vi "getDataByName.vi"(2 "Data Entry Name":string, 3 "Property Array In":T1[](array[typedef])) -> (0 "Value":string[](array[string]), 1 "Entity Type":string[](array[string]))   [LabVIEW 2016]
uses:
  typeDefs/singleDXFobject.ctl
  typeDefs/singleDXFvar.ctl
  dxf typedef.lvlib
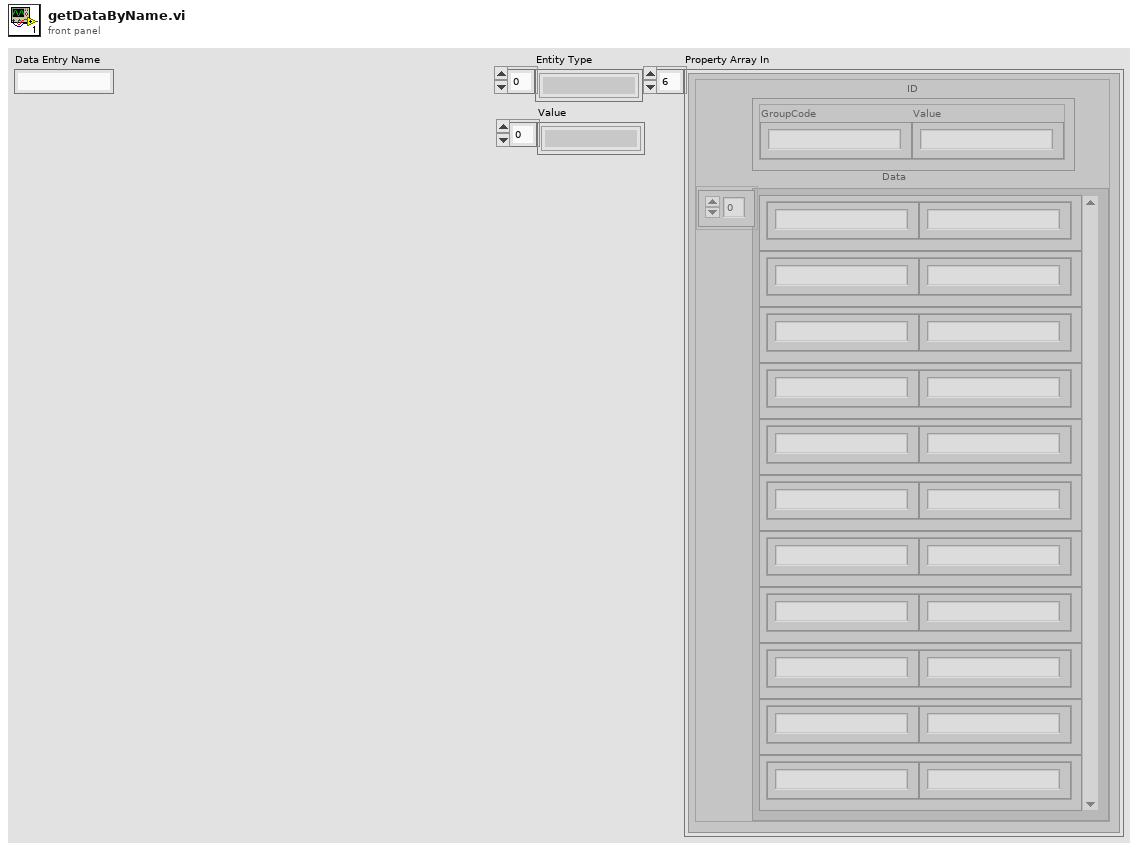
[diagram p1: front panel]
types:
  T1 = typedef "dxf typedef.lvlib/singleDXFobject.ctl" = cluster{"ID":T2, "Data":T2[]}
  T2 = typedef "dxf typedef.lvlib/singleDXFvar.ctl" = cluster{"GroupCode":string, "Value":string}
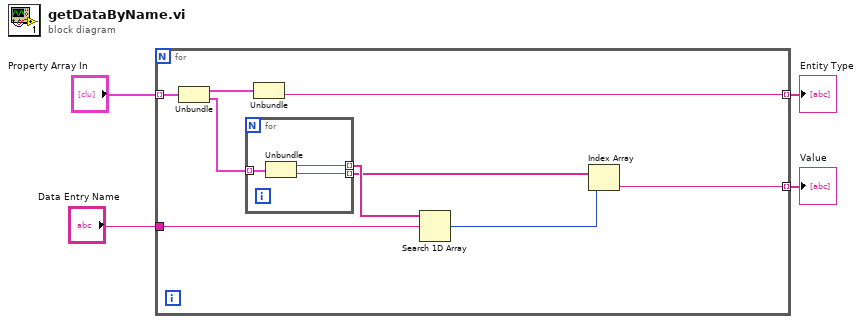
[diagram p0: block diagram]
diagram:
  n1 = for {
    tunnel: "Property Array In" -> [w13] mode=indexing
    tunnel: [w11] -> w3 mode=indexing
    tunnel: "Data Entry Name" -> [w8]
    tunnel: [w5] -> w1 mode=indexing
    n2 = Unbundle(w13) -> ("ID"=w12:T2, "Data"=w10:T2[])
    n3 = for {
      tunnel: w10 -> [w16] mode=indexing
      tunnel: [w15] -> w9 mode=indexing
      tunnel: [w14] -> w7 mode=indexing
      n4 = Unbundle(w16) -> ("GroupCode"=w15:string, "Value"=w14:string)
    }
    n5 = Unbundle(w12) -> ("Value"=w11:string)  [unwired: 1 out]
    n6 = Search 1D Array(1D array=w9, element=w8) -> (index of element=w6:i32)  [unwired: 1 in]
    n7 = Index Array(array=w7, index=w6) -> (element=w5:string)
  }
  "Entity Type" <- w3
  "Value" <- w1
